vi "read_wav.vi"() -> ()   [LabVIEW 2017]
uses:
  <vilib>/rvi/interface/RandomDataEmulation/nirviRandomDataOpen.vi
  <vilib>/rvi/interface/common/niFpgaCacheSessionInfoDynamic.vi
  <vilib>/Utility/error.llb/Error Cluster From Error Code.vi
  <vilib>/rvi/errors/niLvFpgaAdjustHostInterfaceError.vi
  <vilib>/rvi/interface/common/niFpgaWaitOnOcc.vi
  <vilib>/rvi/interface/nirviOpenFPGA/nirviOpenFPGA.xnode
  filter.vi
  <vilib>/rvi/interface/nirviMethod/nirviMethod.xnode
  <vilib>/rvi/errors/niLvFpgaMergeErrorWithErrorCode.vi
  <vilib>/FPGAPlugInAG/Dynamic/niLvFpga_ReadFifo_Dynamic.vi
  <vilib>/FPGAPlugInAG/Dynamic/niLvFpga_WriteFifo_Dynamic.vi
  <vilib>/FPGAPlugInAG/Dynamic/niLvFpga_ConfigureFifo_Dynamic.vi
panel:
  out "DOWNstream":sgl[](graph)=[-3.1872559]
  out "sample rate":dbl
  out "Progress":dbl(slide) scale=0.0..1.0
  out "DMA buffer":i32(slide) scale=0.0..1024.0
  in  "File to upload":path=path "C:/Users/kanaljen/OneDrive - Mälardalens högskola/Robotik III/DVA452/LabVIWE FIFO/mixed.wav"
  out "dt":dbl format="%#_6f s"
  out "Original Signal":waveform(dbl)(graph)={"t0"=timestamp(0 s since 1904-01-01), "dt"=2.2675736961451248e-05, "Y"=array[219309 elements]}
  out "UPstream":dbl(graph)=0.7384033203125
  # "Upload"
  # "Download"
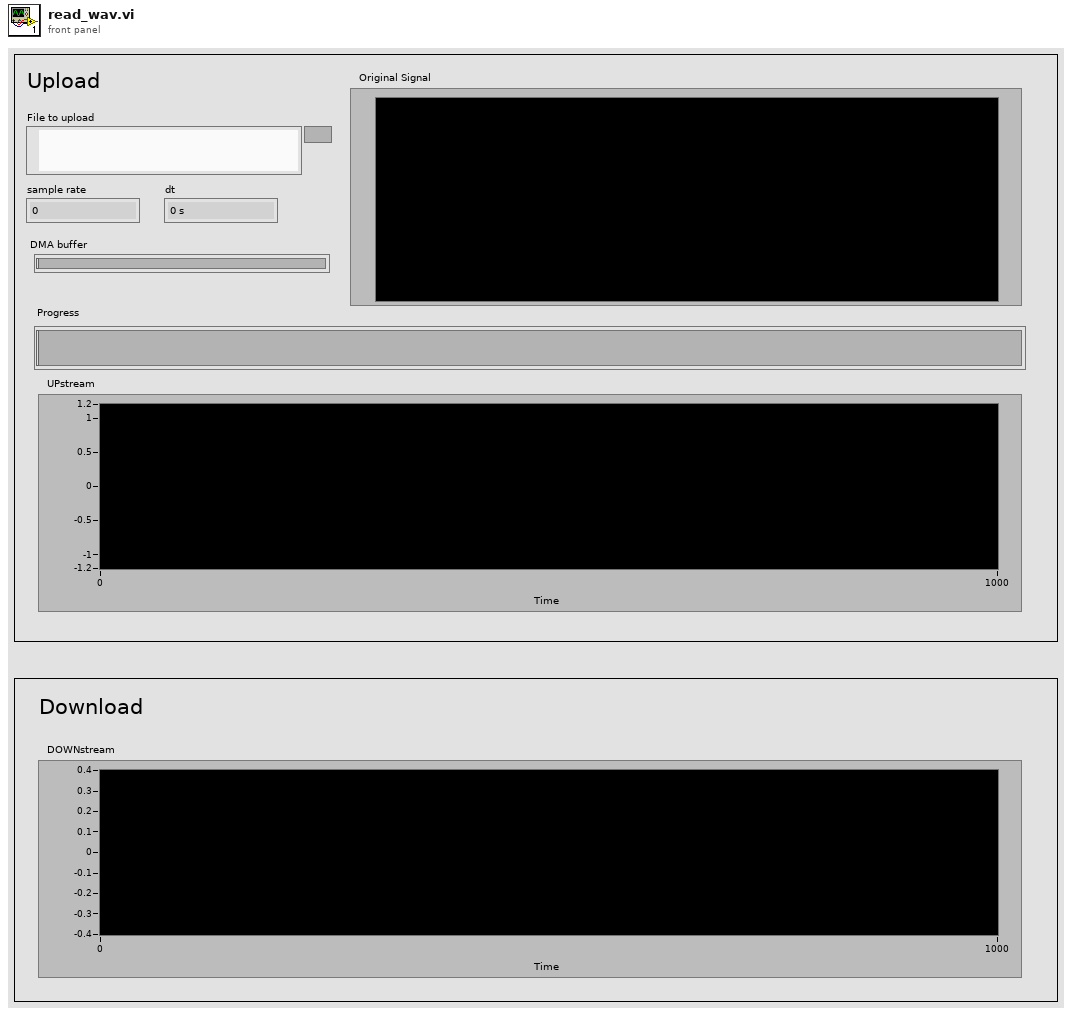
[diagram p1: front panel]
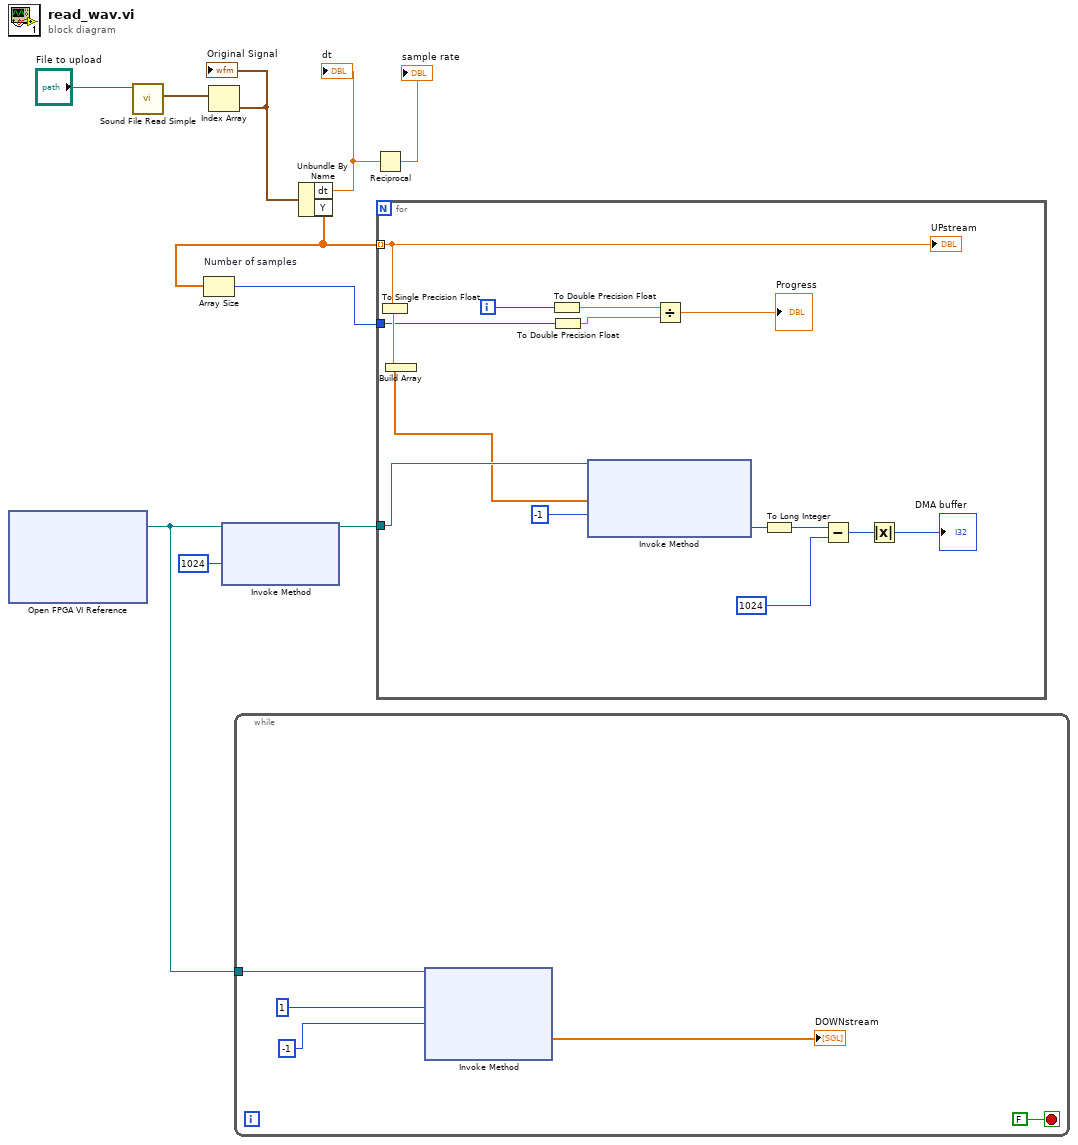
[diagram p0: block diagram]
diagram:
  n1 = xnode "Open FPGA VI Reference"() -> ("FPGA VI Reference Out"=w3:refnum<k20>)  [unwired: 2 in, 1 out]
  n2 = call <vilib>:"Sound File Read Simple.vi"("path"="File to upload") -> ("data"=w6:waveform(dbl)[])  [unwired: 7 in, 3 out]
  n3 = Index Array(array=w6) -> (element=w10:waveform(dbl))  [unwired: 1 in]
  "Original Signal" <- w10
  n4 = xnode "Invoke Method"("FPGA VI Reference In"=w3, "Requested Depth"=1024) -> ("FPGA VI Reference Out"=w1:refnum<k20>)  [unwired: 1 in, 2 out]
  n5 = while {
    tunnel: w3 -> [w14]
    stop <- FALSE stop-if-true
    n6 = xnode "Invoke Method"("FPGA VI Reference In"=w14, "Number of Elements"=1, "Timeout (ms)"=-1) -> ("Data"=→"DOWNstream":sgl[])  [unwired: 1 in, 3 out]
  }
  n7 = Unbundle By Name(w10) -> ("dt"=w5:dbl, "Y"=w9:dbl[])
  "dt" <- w5
  n8 = Array Size "Number of samples"(array=w9) -> (size(s)=w8:i32)
  n9 = Reciprocal(x=w5) -> (1/x=→"sample rate":dbl)
  n10 = for {
    tunnel: w9 -> [w28] mode=indexing
    tunnel: w1 -> [w30]
    tunnel: w8 -> [w17]
    i -> [w19]
    n11 = To Single Precision Float(number=w28) -> (single precision float=w27:sgl)
    n12 = Build Array(w27) -> (w26:sgl[])
    n13 = To Double Precision Float(number=w19) -> (double precision float=w18:dbl)
    n14 = To Double Precision Float(number=w17) -> (double precision float=w16:dbl)
    n15 = xnode "Invoke Method"("FPGA VI Reference In"=w30, "Data"=w26, "Timeout (ms)"=-1) -> ("Empty Elements Remaining"=w23:u32)  [unwired: 1 in, 2 out]
    n16 = Divide(x=w18, y=w16) -> (x/y=→"Progress":dbl)
    n17 = To Long Integer(number=w23) -> (32bit integer=w22:i32)
    n18 = Subtract(x=w22, y=1024) -> (x-y=w21:i32)
    n19 = Absolute Value(x=w21) -> (abs(x)=→"DMA buffer":i32)
    "UPstream" <- w28
  }
